vi "Accelration Control (by Throttle).vi"(2 "acc":dbl, 3 "Yinput":dbl, 4 "Xinput":dbl) -> (0 "Youtput":dbl format="%.2f", 1 "Xoutput":dbl format="%.2f")   [LabVIEW 2015]
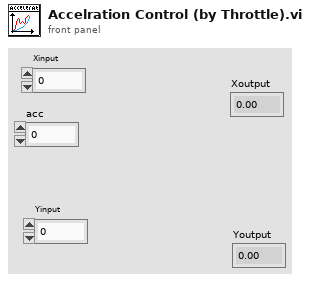
[diagram p1: front panel]
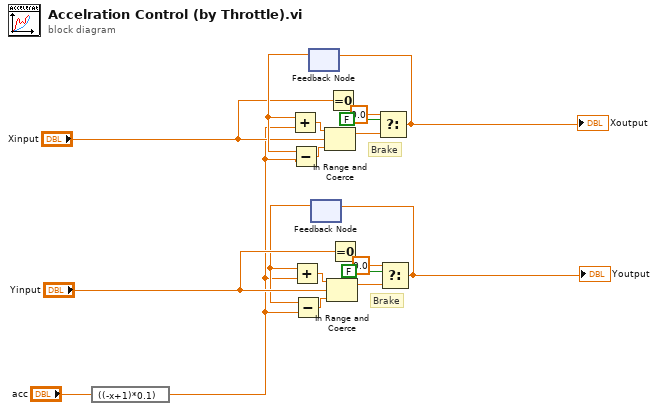
[diagram p0: block diagram]
diagram:
  # "Brake"
  # "Brake"
  n1 = expression code="((-x+1)*0.1)"("acc") -> (w3:dbl)
  n2 = feedback #1() -> (w16:dbl)  [unwired: 1 in]
  n3 = Add(x=w16, y=w3) -> (x+y=w17:dbl)
  n4 = Subtract(x=w16, y=w3) -> (x-y=w18:dbl)
  n5 = feedback #2() -> (w6:dbl)  [unwired: 1 in]
  n6 = Add(x=w6, y=w3) -> (x+y=w5:dbl)
  n7 = Subtract(x=w6, y=w3) -> (x-y=w4:dbl)
  n8 = In Range and Coerce(upper limit=w17, x="Xinput", lower limit=w18) -> (coerced(x)=w13:dbl)  [unwired: 1 out]
  n9 = In Range and Coerce(upper limit=w5, x="Yinput", lower limit=w4) -> (coerced(x)=w8:dbl)  [unwired: 1 out]
  n10 = Equal To 0?(x="Xinput") -> ()  [unwired: 1 out]
  n11 = Equal To 0?(x="Yinput") -> ()  [unwired: 1 out]
  n12 = Select(t=0.0, s=FALSE, f=w13) -> (s? t:f=w11:dbl)
  "Xoutput" <- w11
  n13 = feedback-in #1(w11) -> ()
  n14 = Select(t=0.0, s=FALSE, f=w8) -> (s? t:f=w10:dbl)
  "Youtput" <- w10
  n15 = feedback-in #2(w10) -> ()
